vi "Set_Sweep_Mode_Parameters.vi"(6 "Start mode":i32(ring) items=["Normal", "Waiting for Trigger"], 7 "Sweep Mode":i32(ring) items=["Step one way", "Continuous one way", "Step round trip", "Continuous round trip"], 8 "error in (no error)":errorcluster, 9 "Trigger input":i32(ring) items=["Disable", "Enable"], 10 "Trigger output":i32(ring) items=["None", "Stop", "Start", "Step"], 11 ".NET Reference in":refnum<k24>) -> (0 "error out":errorcluster, 3 "Reference out":refnum<k24>)   [LabVIEW 2017]
uses:
  C:/Users/Ssantec_Test/Documents/Instrument_DLL_Sample_Labview_20220902_Ver1.2.2/DLL/x86/InstrumentDLL.dll
  DLL/x86/InstrumentDLL.dll
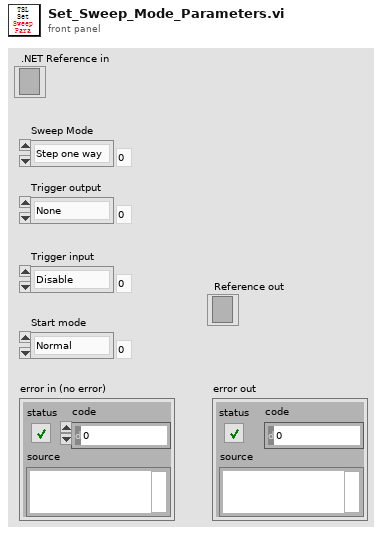
[diagram p1: front panel]
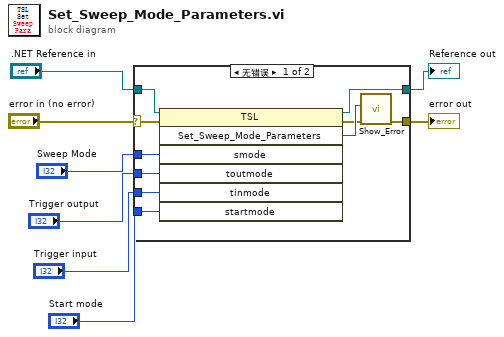
[diagram p0: block diagram]
diagram:
  n1 = case shown="无错误" "error in (no error)" {
    selector: "error in (no error)" -> [w10 w19]
    tunnel: ".NET Reference in" -> [w9 w20]
    tunnel: "Trigger input" -> [w18 _]
    tunnel: "Start mode" -> [w17 _]
    tunnel: "Trigger output" -> [w16 _]
    tunnel: "Sweep Mode" -> [w15 _]
    tunnel: [w14 w20] -> w3
    tunnel: [w11 w19] -> w2
    frame No Error {
      n2 = invoke on="调用节点" class="TSL" method="Set_Sweep_Mode_Parameters"(reference=w9, error in=w10, "smode"=w15, "toutmode"=w16, "tinmode"=w18, "startmode"=w17) -> (reference out=w14:refnum<k24>, error out=w12:errorcluster, "Set_Sweep_Mode_Parameters"=w13:i32)  [unwired: 1 in, 4 out]
      n3 = call "Show_Error.vi"("error in (no error)"=w12, "Error"=w13) -> ("error out"=w11:errorcluster)  [unwired: 9 in]
    }
    frame Error {
    }
  }
  "Reference out" <- w3
  "error out" <- w2
